vi "Write quoted string.vi"(10 "quoted string":bool, 11 "StringFormatter in":refnum<class "StringFormatter.lvclass">) -> (3 "StringFormatter out":refnum<class "StringFormatter.lvclass">)   [LabVIEW 2013, in "OpenStringFormatter.lvlib" / "StringFormatter.lvclass"]
uses:
  StringFormatter.lvclass
  StringFormatter.lvclass/StringFormatter.ctl
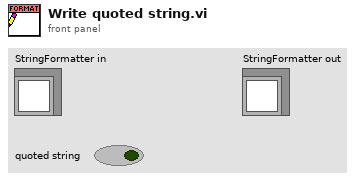
[diagram p1: front panel]
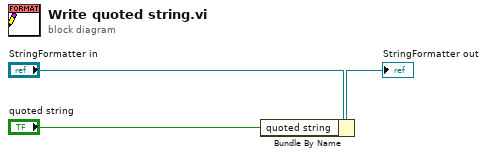
[diagram p0: block diagram]
diagram:
  n1 = Bundle By Name(cluster="StringFormatter in", "quoted string"="quoted string") -> (→"StringFormatter out":refnum<class "StringFormatter.lvclass">)
